vi "Configure_single_trigger.vi"(8 "error in (no error)":errorcluster, 11 "Initialize_card in":refnum<class "Initialize_card.lvclass">) -> (0 "error out":errorcluster, 3 "Initialize_card out":refnum<class "Initialize_card.lvclass">)   [LabVIEW 2015, in "Initialize_card.lvclass"]
uses:
  Initialize_card.lvclass
panel:
  out "Error Code":i32
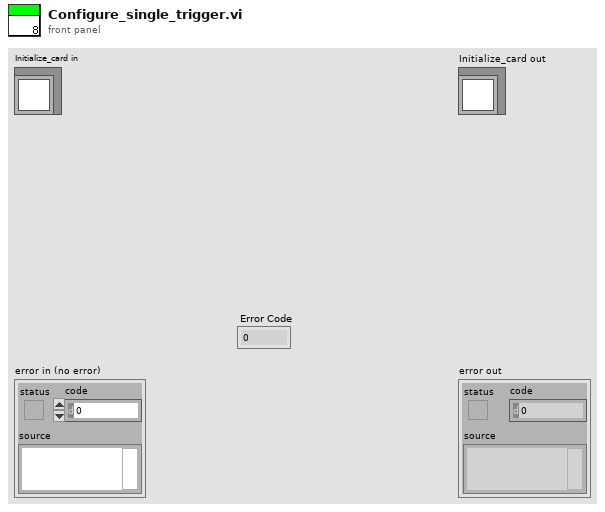
[diagram p1: front panel]
types:
  T1 = cluster{"Handle":u32, "Sample size":u32, "Resolution":i32, "Offset":i32, "Channels":u32, "Boards":u32}
  T2 = cluster{"Slope":u16, "Level":i32, "Source":i32, "External Range":u32, "External Coupling":u16, "External":bool, "Disable":bool, "External Impedance":u16}
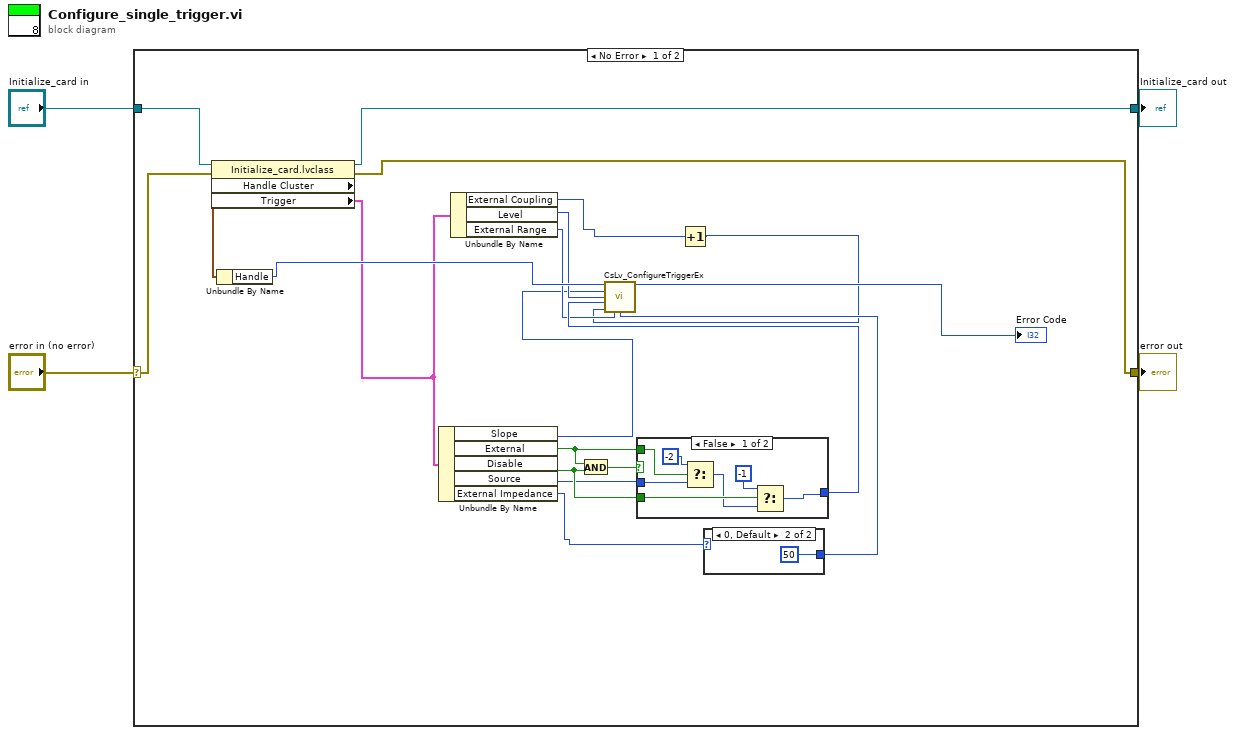
[diagram p0: block diagram]
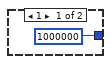
[diagram p2: hidden frame]
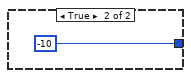
[diagram p3: hidden frame]
diagram:
  n1 = case shown="No Error" "error in (no error)" {
    selector: "error in (no error)" -> [w21 w36]
    tunnel: [w20 w36] -> w3
    tunnel: [w22 w35] -> w1
    tunnel: "Initialize_card in" -> [w23 w35]
    frame No Error {
      n2 = property class="Initialize_card.lvclass"(reference=w23, error in=w21) -> (reference out=w22:refnum<class "Initialize_card.lvclass">, error out=w20:errorcluster, "Handle Cluster"=w19:T1, "Trigger"=w10:T2)
      n3 = Unbundle By Name(w19) -> ("Handle"=w24:u32)
      n4 = Unbundle By Name(w10) -> ("Slope"=w6:u16, "External"=w17:bool, "Disable"=w16:bool, "Source"=w15:i32, "External Impedance"=w5:u16)
      n5 = Unbundle By Name(w10) -> ("External Coupling"=w8:u16, "Level"=w14:i32, "External Range"=w12:u32)
      n6 = And(x=w17, y=w16) -> (x .and. y?=w18:bool)
      n7 = case shown="False" w18 {
        tunnel: [w27 -10] -> w13
        tunnel: w17 -> [w33 _]
        tunnel: w16 -> [w31 _]
        tunnel: w15 -> [w30 _]
        frame False {
          n8 = Select(t=-2, s=w33, f=w30) -> (s? t:f=w28:i32)
          n9 = Select(t=-1, s=w31, f=w28) -> (s? t:f=w27:i32)
        }
        frame True {
        }
      }
      n10 = Increment(x=w8) -> (x+1=w7:u16)
      n11 = case shown="0, Default" w5 {
        tunnel: [u32 1000000 u32 50] -> w11
        frame 1 {
        }
        frame 0, Default {
        }
      }
      n12 = call <userlib>:"CsLv_ConfigureTriggerEx.vi"("Handle"=w24, "Slope (1)"=w6, "Level (0)"=w14, "Source (0)"=w13, "Ext. Coupling (1)"=w7, "External Range (2000 mV)"=w12, "External Impedance (1 MOhm)"=w11) -> ("Error Code"=→"Error Code":i32)  [unwired: 8 in]
    }
    frame Error {
    }
  }
  "error out" <- w3
  "Initialize_card out" <- w1
